vi "Configure Settings.vi"   [LabVIEW 2017]
uses:
  acquisition/Acquisition Settings.ctl
  acquisition/Acquisition State.ctl
  libs/CSV Reader/Mode CSV reader.ctl
  logging/Logging Configuration.ctl
  logging/Logging State.ctl
  libs/PMU Buffer/Buffer Settings.ctl
  processing/Processing Settings.ctl
  2a34ae97-60f5-4341-84c9-4d8c7df74f18.vi
  3968f581-f6d6-4989-85de-0e430d724e00.vi
  38842cf4-451f-4579-bb41-44dc6a1ccd67.vi
  8eb40251-70cd-4357-b466-147393c2f03b.vi
  a47746fd-76d0-4c2d-aaac-f7d470606d9a.vi
  290ce276-0645-466b-8e97-8b13ac2f5f93.vi
  Get Config File Path.vi
  <vilib>/Utility/xml.llb/Read From XML File.vi
  <vilib>/Utility/xml.llb/Read From XML File(string).vi
  <vilib>/Utility/xml.llb/Write to XML File.vi
  <vilib>/Utility/xml.llb/Write to XML File(string).vi
  acquisition/Acquisition.lvlib
  libs/PMU Buffer/PMU data buffer.lvlib
  logging/Logging.lvlib
  processing/Processing.lvlib
  Settings Dialog.vi
  Settings.lvlib
panel:
  # "RUN this VI to load the current settings into the settings dialog, edit them and save them on disk"
types:
  T1 = typedef "Processing.lvlib/Processing Settings.ctl" = cluster{"Settings":string, "Parameters":T2, "Refresh Rate":u32}
  T2 = typedef "PMU data buffer.lvlib/Buffer Settings.ctl" = cluster{"Index":i32, "Size":i32, "Samples":i32, "Ordered ?":bool}
  T3 = typedef "Logging.lvlib/Logging Configuration.ctl" = cluster{"Logging State":T4, "Settings":string, "Buffer":T2}
  T4 = typedef "Logging.lvlib/Logging State.ctl" = enum16{"Idle", "Logging"}
  T5 = typedef "Acquisition.lvlib/Acquisition Settings.ctl" = cluster{"State":T6, "Settings":string, "Online":bool, "S3DK":cluster{"Signals":cluster{"Phasor":string[], "Analog":string[], "Digital":string[]}}, "CSV":cluster{"Index":i32, "Parcel Length":i32, "EOF?":bool, "Config":cluster{"Mode":T7, "delimiter (\\t)":string, "Path":path, "Rectangular?":bool}}}
  T6 = typedef "Acquisition.lvlib/Acquisition State.ctl" = enum16{"Idle", "Idle S3DK", "Acquiring S3DK", "Idle CSV", "Acquiring CSV"}
  T7 = typedef "Mode CSV reader.ctl" = enum16{"Full timestamp", "Relative Time", "Seconds Time", "Nanoseconds Time"}
  T8 = cluster{"Settings Out":T5, "Settings Out":T3, "Settings Out":T1}
  T9 = typedef "Settings.lvlib/Settings.ctl" = cluster{"Acquisition":T5, "Logging":T3, "Processing":T1}
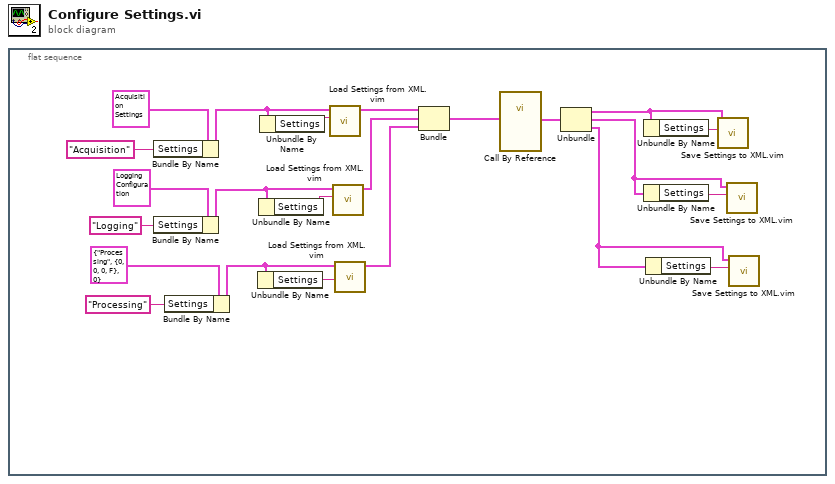
[diagram p0: block diagram]
diagram:
  n1 = flat-sequence {
    frame #0 {
      n2 = Bundle By Name(cluster=T5 {"State"=enum."Idle S3DK", "Settings"="Acquisition", "Online"=FALSE, "S3DK"={"Signals"={"Phasor"=[], "Analog"=[], "Digital"=[]}}, "CSV"={"Index"=0, "Parcel Length"=0, "EOF?"=FALSE, "Config"={"Mode"=enum."Full timestamp", "delimiter (\\t)"="\t", "Path"=path "", "Rectangular?"=FALSE}}} ("Data Cluster"), "Settings"="Acquisition") -> (w17:T5)
      n3 = Bundle By Name(cluster=T3 {"Logging State"=enum."Idle", "Settings"="Logging", "Buffer"={"Index"=0, "Size"=15000, "Samples"=0, "Ordered ?"=FALSE}} ("Logging Configuration"), "Settings"="Logging") -> (w15:T3)
      n4 = Bundle By Name(cluster=T1 {"Settings"="Processing", "Parameters"={"Index"=0, "Size"=0, "Samples"=0, "Ordered ?"=FALSE}, "Refresh Rate"=0} ("Processing Settings"), "Settings"="Processing") -> (w13:T1)
      n5 = Unbundle By Name(w13) -> ("Settings"=w12:string)
      n6 = Unbundle By Name(w15) -> ("Settings"=w14:string)
      n7 = Unbundle By Name(w17) -> ("Settings"=w16:string)
      n8 = call "Load Settings from XML.vim"("Settings File Name"=w16, "Settings In"=w17) -> ("Settings Out"=w11:T5)  [unwired: 8 in, 1 out]
      n9 = call "Load Settings from XML.vim"("Settings File Name"=w14, "Settings In"=w15) -> ("Settings Out"=w10:T3)  [unwired: 8 in, 1 out]
      n10 = call "Load Settings from XML.vim"("Settings File Name"=w12, "Settings In"=w13) -> ("Settings Out"=w9:T1)  [unwired: 8 in, 1 out]
      n11 = Bundle("Settings Out"=w11, "Settings Out"=w10, "Settings Out"=w9) -> (w8:T8)  [unwired: 1 in]
      n12 = call-by-ref "?"("Settings in"=w8) -> ("Settings out"=w6:T9)  [unwired: 9 in, 5 out]
      n13 = Unbundle(w6) -> ("Acquisition"=w3:T5, "Logging"=w2:T3, "Processing"=w1:T1)
      n14 = Unbundle By Name(w3) -> ("Settings"=w7:string)
      n15 = Unbundle By Name(w2) -> ("Settings"=w5:string)
      n16 = Unbundle By Name(w1) -> ("Settings"=w4:string)
      n17 = call "Save Settings to XML.vim"("Settings File Name"=w7, "Settings In"=w3) -> ()  [unwired: 9 in, 1 out]
      n18 = call "Save Settings to XML.vim"("Settings File Name"=w5, "Settings In"=w2) -> ()  [unwired: 9 in, 1 out]
      n19 = call "Save Settings to XML.vim"("Settings File Name"=w4, "Settings In"=w1) -> ()  [unwired: 9 in, 1 out]
    }
  }
